vi "Multiplexer_MeasurementAndControl.vi"(8 "error in (no error)":errorcluster, 10 "Multiplexer_Cluser":T1, 11 "Task in":refnum<k21>) -> (0 "error out":errorcluster, 2 "Data_Array":dbl[](array[numeric]), 3 "Task out":refnum<k21>)   [LabVIEW 2020]
uses:
  <vilib>/DAQmx/read.llb/DAQmx Read (Analog 1D DBL NChan 1Samp).vi
  <vilib>/DAQmx/miscellaneous.llb/DAQmx Fill In Error Info.vi
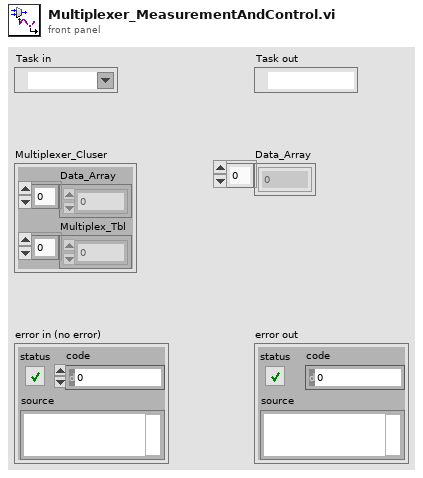
[diagram p1: front panel]
types:
  T1 = cluster{"Data_Array":dbl[], "Multiplex_Tbl":u32[]}
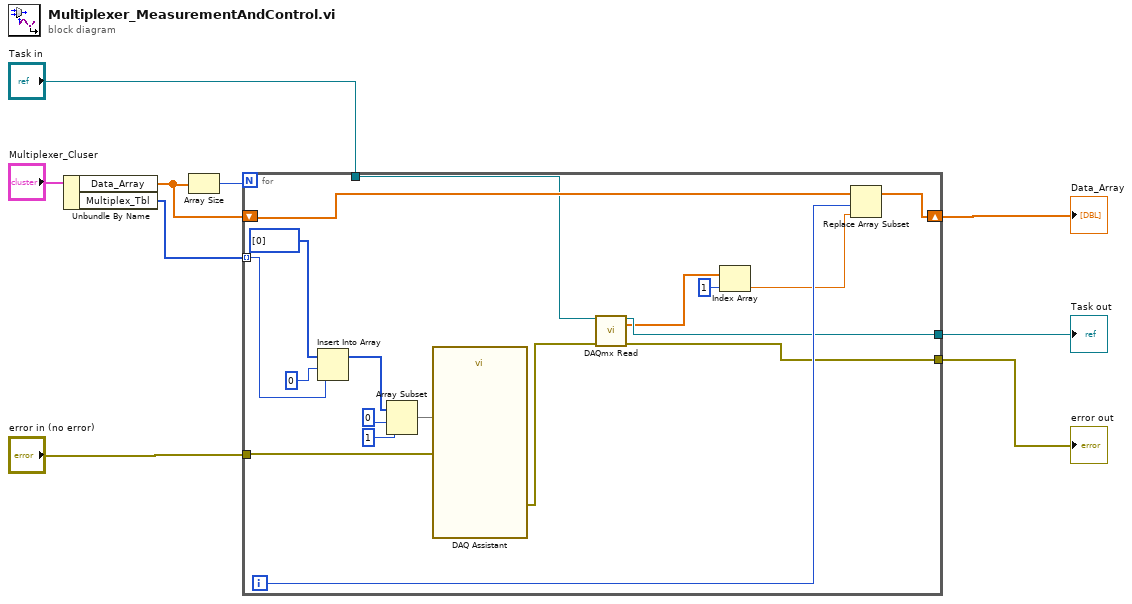
[diagram p0: block diagram]
diagram:
  n1 = Unbundle By Name("Multiplexer_Cluser") -> ("Data_Array"=w3:dbl[], "Multiplex_Tbl"=w6:u32[])
  n2 = Array Size(array=w3) -> (size(s)=w2:i32)
  n3 = for {
    N: w2 -> [_]
    shift-right: [w14] -> w5
    shift-left: w3 -> [w27]
    tunnel: "error in (no error)" -> [w26]
    tunnel: w6 -> [w23] mode=indexing
    tunnel: "Task in" -> [w17]
    tunnel: [w16] -> w8
    tunnel: [w15] -> w9
    i -> [w24]
    n4 = Insert Into Array(array=u32[] [0] ("data"), index=0, new element=w23) -> (w19:u32[])
    n5 = Array Subset(array=w19, index=0, length=1) -> (w18:u32[])
    n6 = call "DAQ Assistant"("data"=w18, "error in"=w26) -> ("error out"=w10:errorcluster)  [unwired: 16 in, 1 out]
    n7 = call-poly <vilib>:"DAQmx Read.vi"("task/channels in"=w17, "error in"=w10) -> ("task out"=w16:refnum<k21>, "data"=w13:dbl[], "error out"=w15:errorcluster)  [unwired: 11 in]
    n8 = Index Array(array=w13, index=1) -> (element=w11:dbl)
    n9 = Replace Array Subset(array=w27, new element=w11, index=w24) -> (w14:dbl[])
  }
  "error out" <- w9
  "Task out" <- w8
  "Data_Array" <- w5
